vi "addorminus.vi"() -> ()   [LabVIEW 2016]
panel:
  in  "stop":bool
  in  "Boolean":bool
  out "Numeric 3":dbl
  in  "Numeric 2":dbl
  in  "Numeric":dbl
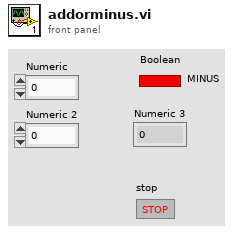
[diagram p1: front panel]
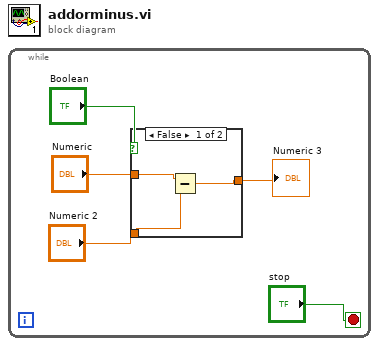
[diagram p0: block diagram]
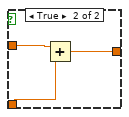
[diagram p2: hidden frame]
diagram:
  n1 = while {
    stop <- "stop" stop-if-true
    n2 = case shown="False" "Boolean" {
      tunnel: "Numeric" -> [w8 w11]
      tunnel: "Numeric 2" -> [w7 w10]
      tunnel: [w6 w9] -> w1
      frame False {
        n3 = Subtract(x=w8, y=w7) -> (x-y=w6:dbl)
      }
      frame True {
        n4 = Add(x=w11, y=w10) -> (x+y=w9:dbl)
      }
    }
    "Numeric 3" <- w1
  }
